vi "Main Page.vi"(8 "error in (no error)":errorcluster, 11 "Node Ptr":T1 format="%.0x") -> (0 "error out":errorcluster)   [LabVIEW 2021, in "DAQ Analog InOut System Explorer.lvlib"]
uses:
  DAQ Analog InOut System Explorer.lvlib
  <vilib>/NI VeriStand/Custom Device API/Custom Device Item Ref.ctl
  <vilib>/NI VeriStand/Custom Device API/Custom Device API.lvlib
panel:
  in  "Configure Physical Channels":bool
  in  "AO Channels Used":u8=1
  in  "AI Channels Used":u8=1
  in  "Select channel type to add":string(combo)
  in  "Device Name in Max":string="PXI1Slot2" caption="Device Name (Ex: PXI1Slot2)"
  in  "PCL Decimation":u16
  in  "Async Timeout (ms)":u16
  out "Version":string
  in  "Specific Header":cluster{"Section Name":string}={"Section Name"="Custom Device Item Settings"}
  in  "General Header":cluster{"Section Name":string}={"Section Name"="General Custom Device Settings"}
  in  "Description":string
  in  "Name":string
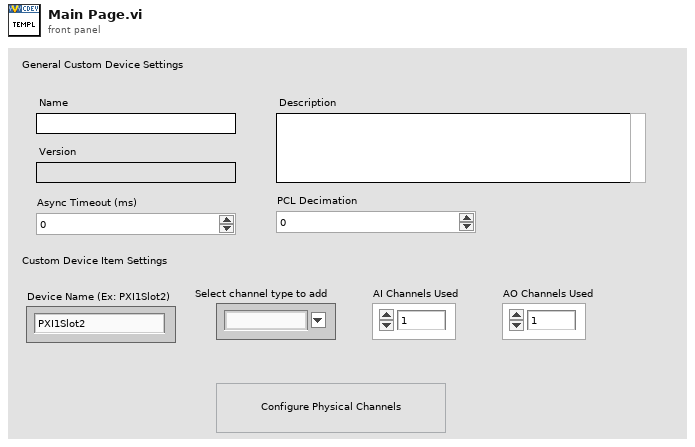
[diagram p1: front panel]
types:
  T1 = typedef "Custom Device API.lvlib/Custom Device Item Ref.ctl" = u64
  T2 = typedef "Custom Device API.lvlib/Custom Device Item Info.ctl" = cluster{"Name":string, "Is Channel":bool, "GUID":string, "Is Waveform":bool}
  T3 = typedef "DAQ Analog InOut System Explorer.lvlib/Main Page Parameters.ctl" = cluster{"AI Channels Used":u8, "AO Channels Used":u8, "Select channel type to add":string, "Device Name in Max":string, "PCL Decimation":u16, "Async Timeout (ms)":u16}
  T4 = typedef "Custom Device API.lvlib/Custom Device Commands.ctl" = enum16{"Default", "Item renamed", "Shutdown", "Dynamic button pressed"}
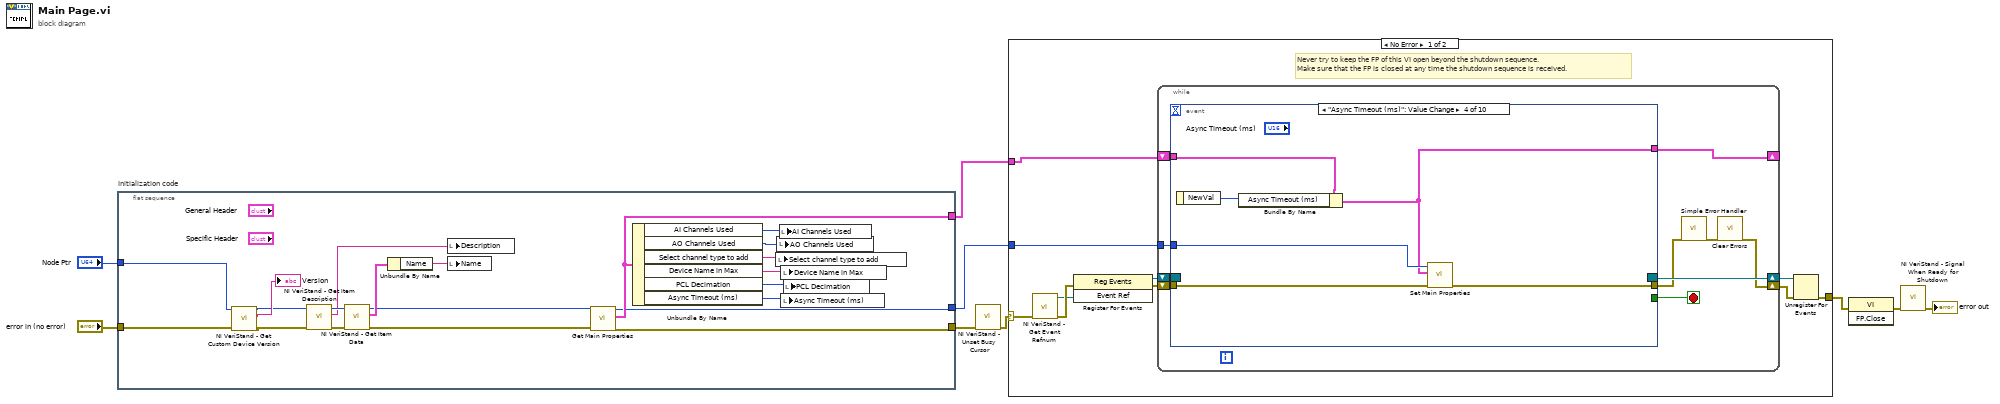
[diagram p0: block diagram]
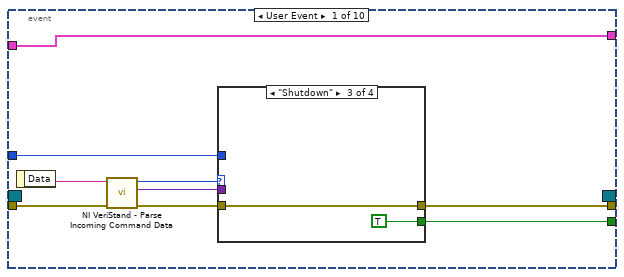
[diagram p2: hidden frame]
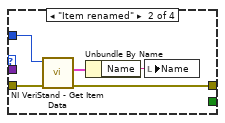
[diagram p4: hidden frame]
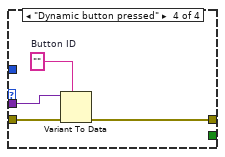
[diagram p5: hidden frame]
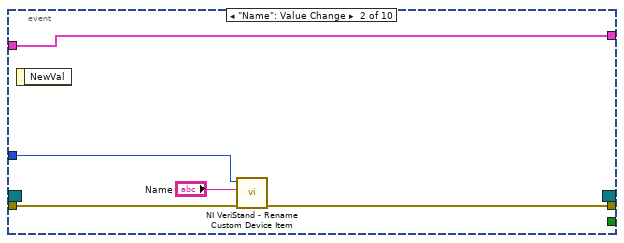
[diagram p6: hidden frame]
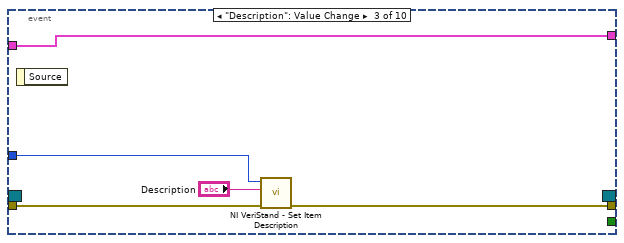
[diagram p7: hidden frame]
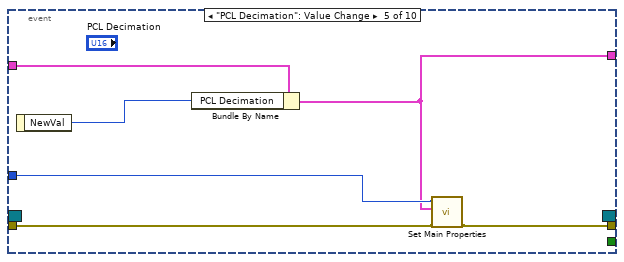
[diagram p8: hidden frame]
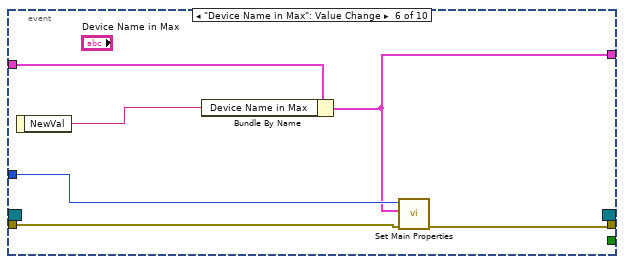
[diagram p9: hidden frame]
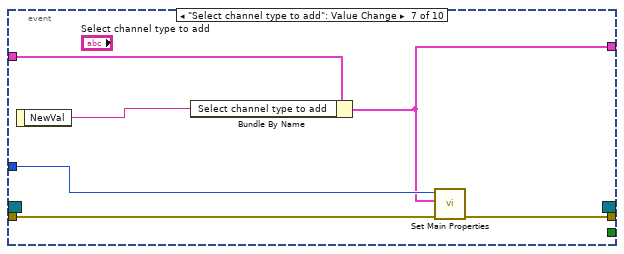
[diagram p10: hidden frame]
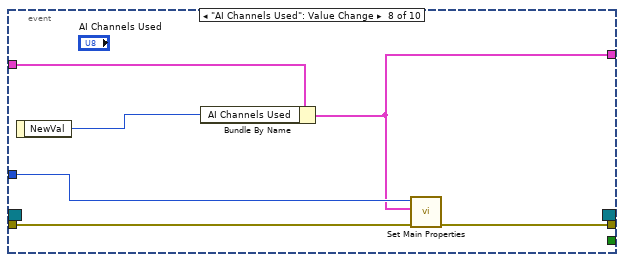
[diagram p11: hidden frame]
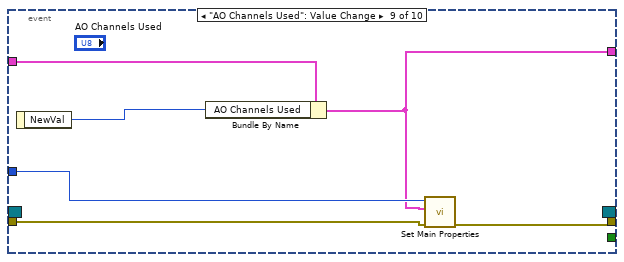
[diagram p12: hidden frame]
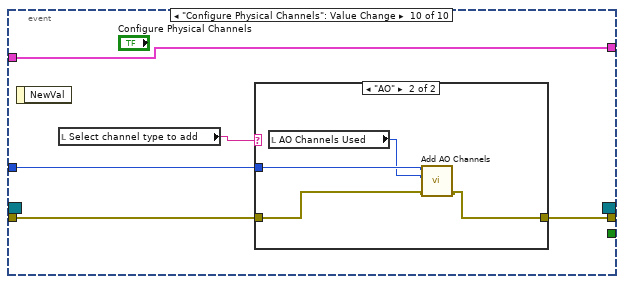
[diagram p13: hidden frame]
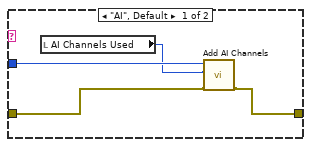
[diagram p14: hidden frame]
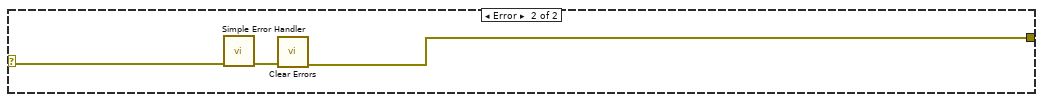
[diagram p15: hidden frame]
diagram:
  n1 = flat-sequence "Initialization code" {
    tunnel: "error in (no error)" -> [w17]
    tunnel: "Node Ptr" -> [w21]
    tunnel: [w24] -> w5
    tunnel: [w22] -> w2
    tunnel: [w23] -> w1
    frame #0 {
      n2 = call <vilib>:"NI VeriStand - Get Custom Device Version.vi"("error in (no error)"=w17, "Device Ref in"=w21) -> ("error out"=w20:errorcluster, "Value"=→"Version":string, "Device Ref out"=w18:T1)  [unwired: 7 in]
      n3 = call <vilib>:"NI VeriStand - Get Item Description.vi"("error in (no error)"=w20, "Item Ref in"=w18) -> ("error out"=w29:errorcluster, "Description"=w26:string, "Item Ref out"=w30:T1)  [unwired: 7 out]
      n4 = call <vilib>:"NI VeriStand - Get Item Data.vi"("error in (no error)"=w29, "Item Ref in"=w30) -> ("error out"=w11:errorcluster, "Item Info"=w28:T2, "Item Ref out"=w10:T1)  [unwired: 7 out]
      n5 = Unbundle By Name(w28) -> ("Name"=w27:string)
      n6 = local write "Description"(w26) -> ()
      n7 = local write "Name"(w27) -> ()
      n8 = call "Get Main Properties.vi"("error in (no error)"=w11, "Ref in"=w10) -> ("error out"=w24:errorcluster, "Main Page Parameters"=w23:T3, "Ref out"=w22:T1)  [unwired: 7 in]
      n9 = Unbundle By Name(w23) -> ("AI Channels Used"=w13:u8, "AO Channels Used"=w14:u8, "Select channel type to add"=w15:string, "Device Name in Max"=w16:string, "PCL Decimation"=w25:u16, "Async Timeout (ms)"=w12:u16)
      n10 = local write "Select channel type to add"(w15) -> ()
      n11 = local write "AO Channels Used"(w14) -> ()
      n12 = local write "AI Channels Used"(w13) -> ()
      n13 = local write "Device Name in Max"(w16) -> ()
      n14 = local write "Async Timeout (ms)"(w12) -> ()
      n15 = local write "PCL Decimation"(w25) -> ()
    }
  }
  n16 = call <vilib>:"NI VeriStand - Unset Busy Cursor.vi"("error in (no error)"=w5) -> ("error out"=w4:errorcluster)  [unwired: 10 out]
  n17 = case shown="No Error" w4 {
    selector: w4 -> [w32 w133]
    tunnel: [w37 w131] -> w9
    tunnel: w2 -> [w33 _]
    tunnel: w1 -> [w31 _]
    frame No Error {
      # "Never try to keep the FP of this VI open beyond the shutdown sequence.\nMake sure that the FP is closed at any time the shutdown sequence is received."
      n18 = call <vilib>:"NI VeriStand - Get Event Refnum.vi"("error in (no error)"=w32) -> ("error out"=w40:errorcluster, "Event Ref"=w36:refnum<user-event>)  [unwired: 9 out]
      n19 = register-events(error in=w40, w36) -> (reference out=w34:refnum<event-registration>, error out=w35:errorcluster)  [unwired: 1 in]
      n20 = while {
        tunnel: w33 -> [w46]
        shift-right: [w43] -> w38
        shift-left: w35 -> [w49]
        shift-right: [w50] -> w39
        shift-left: w34 -> [w48]
        shift-right: [w41] -> _
        shift-left: w31 -> [w42]
        stop <- w47 stop-if-true
        n21 = event shown="[3] \"Async Timeout (ms)\": Value Change" {
          selector: w48 -> [_ _ _ _ _ _ _ _ _ _]
          dyn-events: [_ _ _ _ _ _ _ _ _ _] -> w50
          timeout: _ -> [_ _ _ _ _ _ _ _ _ _]
          tunnel: w49 -> [w59 w76 w80 w86 w89 w95 w101 w107 w113 w120]
          tunnel: [w55 _ _ _ _ _ _ _ _ _] -> w47
          tunnel: [w54 w75 w79 w85 w88 w94 w100 w106 w112 w119] -> w45
          tunnel: w46 -> [w53 w74 w81 w87 w91 w97 w103 w109 w115 w121]
          tunnel: w42 -> [w51 w72 w77 w84 w93 w99 w105 w111 w117 w118]
          tunnel: [w51 w72 w77 w82 w90 w96 w102 w108 w114 w118] -> w41
          event User Event {
            n22 = event-data() -> ("Data"=w58:string)  [unwired: 1 out]
            n23 = call <vilib>:"NI VeriStand - Parse Incoming Command Data.vi"("error in (no error)"=w59, "Incoming data"=w58) -> ("error out"=w57:errorcluster, "Outgoing data"=w52:variant, "Action"=w56:T4)  [unwired: 7 out]
            n24 = case shown="\"Shutdown\"" w56 {
              tunnel: w57 -> [w60 w65 w66 w71]
              tunnel: [_ _ TRUE _] -> w55
              tunnel: [w60 w62 w66 w68] -> w54
              tunnel: w53 -> [_ w64 _ _]
              tunnel: w52 -> [_ _ _ w70]
              frame "Default", Default {
              }
              frame "Item renamed" {
                n25 = call <vilib>:"NI VeriStand - Get Item Data.vi"("error in (no error)"=w65, "Item Ref in"=w64) -> ("error out"=w62:errorcluster, "Item Info"=w63:T2)  [unwired: 8 out]
                n26 = Unbundle By Name(w63) -> ("Name"=w61:string)
                n27 = local write "Name"(w61) -> ()
              }
              frame "Shutdown" {
              }
              frame "Dynamic button pressed" {
                w69 = ""  # Button ID
                n28 = Variant To Data(error in=w71, type=w69, Variant=w70) -> (error out=w68:errorcluster)  [unwired: 1 out]
              }
            }
          }
          event "Name": Value Change {
            n29 = event-data() -> ()  [unwired: 2 out]
            n30 = call <vilib>:"NI VeriStand - Rename Custom Device Item.vi"("error in (no error)"=w76, "New Name"="Name", "Item Ref in"=w74) -> ("error out"=w75:errorcluster)  [unwired: 1 in, 7 out]
          }
          event "Description": Value Change {
            n31 = event-data() -> ()  [unwired: 2 out]
            n32 = call <vilib>:"NI VeriStand - Set Item Description.vi"("error in (no error)"=w80, "Description"="Description", "Item Ref in"=w81) -> ("error out"=w79:errorcluster)  [unwired: 8 out]
          }
          event "Async Timeout (ms)": Value Change {
            n33 = event-data() -> ("NewVal"=w83:u16)  [unwired: 1 out]
            n34 = Bundle By Name(cluster=w84, "Async Timeout (ms)"=w83) -> (w82:T3)
            n35 = call "Set Main Properties.vi"("error in (no error)"=w86, "Main Page Parameters"=w82, "Ref in"=w87) -> ("error out"=w85:errorcluster)  [unwired: 7 in, 1 out]
          }
          event "PCL Decimation": Value Change {
            n36 = event-data() -> ("NewVal"=w92:u16)  [unwired: 1 out]
            n37 = Bundle By Name(cluster=w93, "PCL Decimation"=w92) -> (w90:T3)
            n38 = call "Set Main Properties.vi"("error in (no error)"=w89, "Main Page Parameters"=w90, "Ref in"=w91) -> ("error out"=w88:errorcluster)  [unwired: 7 in, 1 out]
          }
          event "Device Name in Max": Value Change {
            n39 = event-data() -> ("NewVal"=w98:string)  [unwired: 1 out]
            n40 = Bundle By Name(cluster=w99, "Device Name in Max"=w98) -> (w96:T3)
            n41 = call "Set Main Properties.vi"("error in (no error)"=w95, "Main Page Parameters"=w96, "Ref in"=w97) -> ("error out"=w94:errorcluster)  [unwired: 7 in, 1 out]
          }
          event "Select channel type to add": Value Change {
            n42 = event-data() -> ("NewVal"=w104:string)  [unwired: 1 out]
            n43 = Bundle By Name(cluster=w105, "Select channel type to add"=w104) -> (w102:T3)
            n44 = call "Set Main Properties.vi"("error in (no error)"=w101, "Main Page Parameters"=w102, "Ref in"=w103) -> ("error out"=w100:errorcluster)  [unwired: 7 in, 1 out]
          }
          event "AI Channels Used": Value Change {
            n45 = event-data() -> ("NewVal"=w110:u8)  [unwired: 1 out]
            n46 = Bundle By Name(cluster=w111, "AI Channels Used"=w110) -> (w108:T3)
            n47 = call "Set Main Properties.vi"("error in (no error)"=w107, "Main Page Parameters"=w108, "Ref in"=w109) -> ("error out"=w106:errorcluster)  [unwired: 7 in, 1 out]
          }
          event "AO Channels Used": Value Change {
            n48 = event-data() -> ("NewVal"=w116:u8)  [unwired: 1 out]
            n49 = Bundle By Name(cluster=w117, "AO Channels Used"=w116) -> (w114:T3)
            n50 = call "Set Main Properties.vi"("error in (no error)"=w113, "Main Page Parameters"=w114, "Ref in"=w115) -> ("error out"=w112:errorcluster)  [unwired: 7 in, 1 out]
          }
          event "Configure Physical Channels": Value Change {
            n51 = event-data() -> ()  [unwired: 2 out]
            n52 = local read "Select channel type to add"() -> (w122:string)
            n53 = case shown="\"AO\"" w122 {
              tunnel: w121 -> [w126 w130]
              tunnel: w120 -> [w124 w128]
              tunnel: [w123 w127] -> w119
              frame "AI", Default {
                n54 = local read "AI Channels Used"() -> (w125:u8)
                n55 = call "Add AI Channels.vi"("error in (no error)"=w124, "Channels"=w125, "Device Item Ref in"=w126) -> ("error out"=w123:errorcluster)  [unwired: 7 in, 1 out]
              }
              frame "AO" {
                n56 = local read "AO Channels Used"() -> (w129:u8)
                n57 = call "Add AO Channels.vi"("error in (no error)"=w128, "Channels"=w129, "Device Item Ref in"=w130) -> ("error out"=w127:errorcluster)  [unwired: 7 in, 1 out]
              }
            }
          }
        }
        n58 = call <vilib>:"Simple Error Handler.vi"("error in (no error)"=w45) -> ("error out"=w44:errorcluster)  [unwired: 1 in, 7 out]
        n59 = call <vilib>:"Clear Errors.vi"("error in (no error)"=w44) -> ("error out"=w43:errorcluster)  [unwired: 1 in, 5 out]
      }
      n60 = Unregister For Events(event registration refnum=w39, error in=w38) -> (error out=w37:errorcluster)
    }
    frame Error {
      n61 = call <vilib>:"Simple Error Handler.vi"("error in (no error)"=w133) -> ("error out"=w132:errorcluster)  [unwired: 1 in, 7 out]
      n62 = call <vilib>:"Clear Errors.vi"("error in (no error)"=w132) -> ("error out"=w131:errorcluster)  [unwired: 1 in, 5 out]
    }
  }
  n63 = invoke class="VI" method="FP.Close"(error in=w9) -> (error out=w8:errorcluster)  [unwired: 2 in, 2 out]
  n64 = call <vilib>:"NI VeriStand - Signal When Ready for Shutdown.vi"("error in (no error)"=w8) -> ("error out"=→"error out":errorcluster)  [unwired: 10 out]
